vi "dotNETChart_DataChangeEvent.vi"(9 "Chart Settings clstr":T1={"Enable Mouse Zoom (only works in 2D mode)"=TRUE, "Chart Wall Transparency Level"=37, "Chart Wall Colour"=0, "x axis label"="X axis title", "y axis label"="Y axis title", "Enable3D"=TRUE, "3D Settings"={"Inclination"=20, "LightStyle"=2, "Perspective"=4, "WallWidth"=5, "Rotation"=25}, "BackGradientStyle"=2, "SkinStyle"=1, "Chart Background Gradient Colour"=0, "Chart Border Colour"=0, "Palette"=12, "LegendStyle"=0, "ChartType"=[10, 13], "SeriesDataColour"=[]} {"ChartType" items=["Point", "FastPoint", "Bubble", "Line", "Spline", "StepLine", "FastLine", "Bar", "StackedBar", "StackedBar100", "Column", "StackedColumn", "StackedColumn100", "Area", "SplineArea", "StackedArea", "StackedArea100", "Pie", "Doughnut", "Stock", "Candlestick", "Range", "SplineRange", "RangeBar", "RangeColumn", "Radar", "Polar", "ErrorBar", "BoxPlot", "Renko", "ThreeLineBreak", "Kagi", "PointAndFigure", "Funnel", "Pyramid"]; "LegendStyle" items=["Column", "Row", "Table"]; "Palette" items=["None", "Bright", "Grayscale", "Excel", "Light", "Pastel", "EarthTones", "SemiTransparent", "Berry", "Chocolate", "Fire", "SeaGreen", "BrightPastel"]; "SkinStyle" items=["None", "Emboss", "Raised", "Sunken", "FrameThin1", "FrameThin2", "FrameThin3", "FrameThin4", "FrameThin5", "FrameThin6", "FrameTitle1", "FrameTitle2", "FrameTitle3", "FrameTitle4", "FrameTitle5", "FrameTitle6", "FrameTitle7", "FrameTitle8"]; "BackGradientStyle" items=["None", "LeftRight", "TopBottom", "Center", "DiagonalLeft", "DiagonalRight", "HorizontalCenter", "VerticalCenter"]; "3D Settings"."LightStyle" items=["None", "Simplistic", "Realistic"]}, 10 "Microsoft Chart":refnum<k24>, 11 "chart data":dynamicdata(graph) caption="Chart Data") -> (0 "error out":errorcluster, 2 "reference out":refnum<k24>)   [LabVIEW 2013, in "dotNETChart XControl.xctl"]
uses:
  dotNETChart XControl.xctl
  System.Windows.Forms.DataVisualization
  typedefs/ChartSettings cluster.ctl
  typedefs/3DSettings.ctl
  typedefs/BackGradientStyle.ctl
  typedefs/SkinStyle.ctl
  typedefs/Palette.ctl
  typedefs/LegendStyle.ctl
  typedefs/ChartType.ctl
  System.Drawing
  <vilib>/express/express shared/transition.llb/Dynamic To Waveform Array.vi
  <vilib>/express/express signal manip/GetorSetDDTAttributes/Get DDT Attributes/Get DDT Properties.xnode
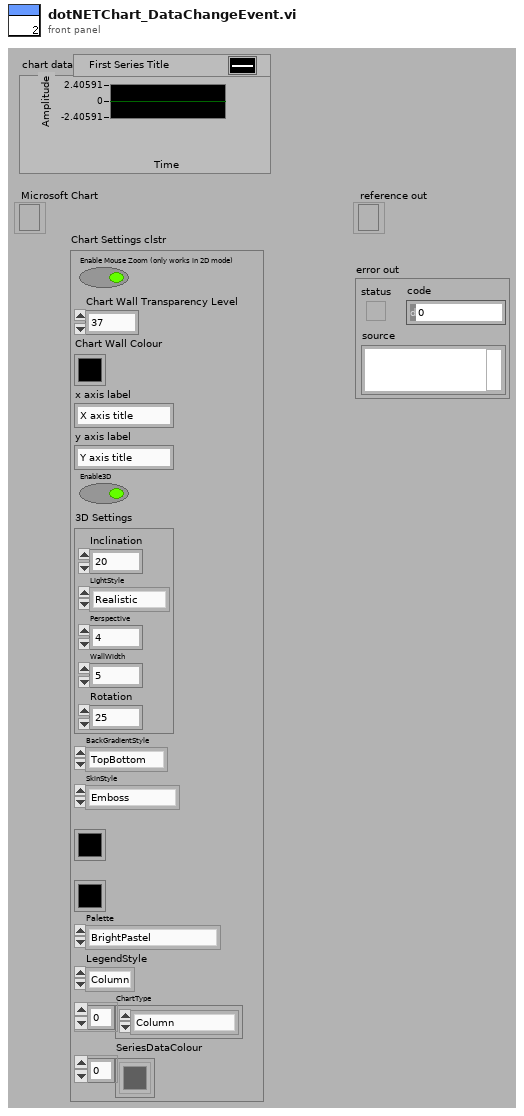
[diagram p1: front panel]
types:
  T1 = typedef "ChartSettings cluster.ctl" = cluster{"Enable Mouse Zoom (only works in 2D mode)":bool, "Chart Wall Transparency Level":i32, "Chart Wall Colour":u32, "x axis label":string, "y axis label":string, "Enable3D":bool, "3D Settings":T2, "BackGradientStyle":T3, "SkinStyle":T4, "Chart Background Gradient Colour":u32, "Chart Border Colour":u32, "Palette":T5, "LegendStyle":T6, "ChartType":T7[], "SeriesDataColour":u32[]}
  T2 = typedef "3DSettings.ctl" = cluster{"Inclination":i32, "LightStyle":i32, "Perspective":i32, "WallWidth":i32, "Rotation":i32}
  T3 = typedef "BackGradientStyle.ctl" = i32
  T4 = typedef "SkinStyle.ctl" = i32
  T5 = typedef "Palette.ctl" = i32
  T6 = typedef "LegendStyle.ctl" = i32
  T7 = typedef "ChartType.ctl" = i32
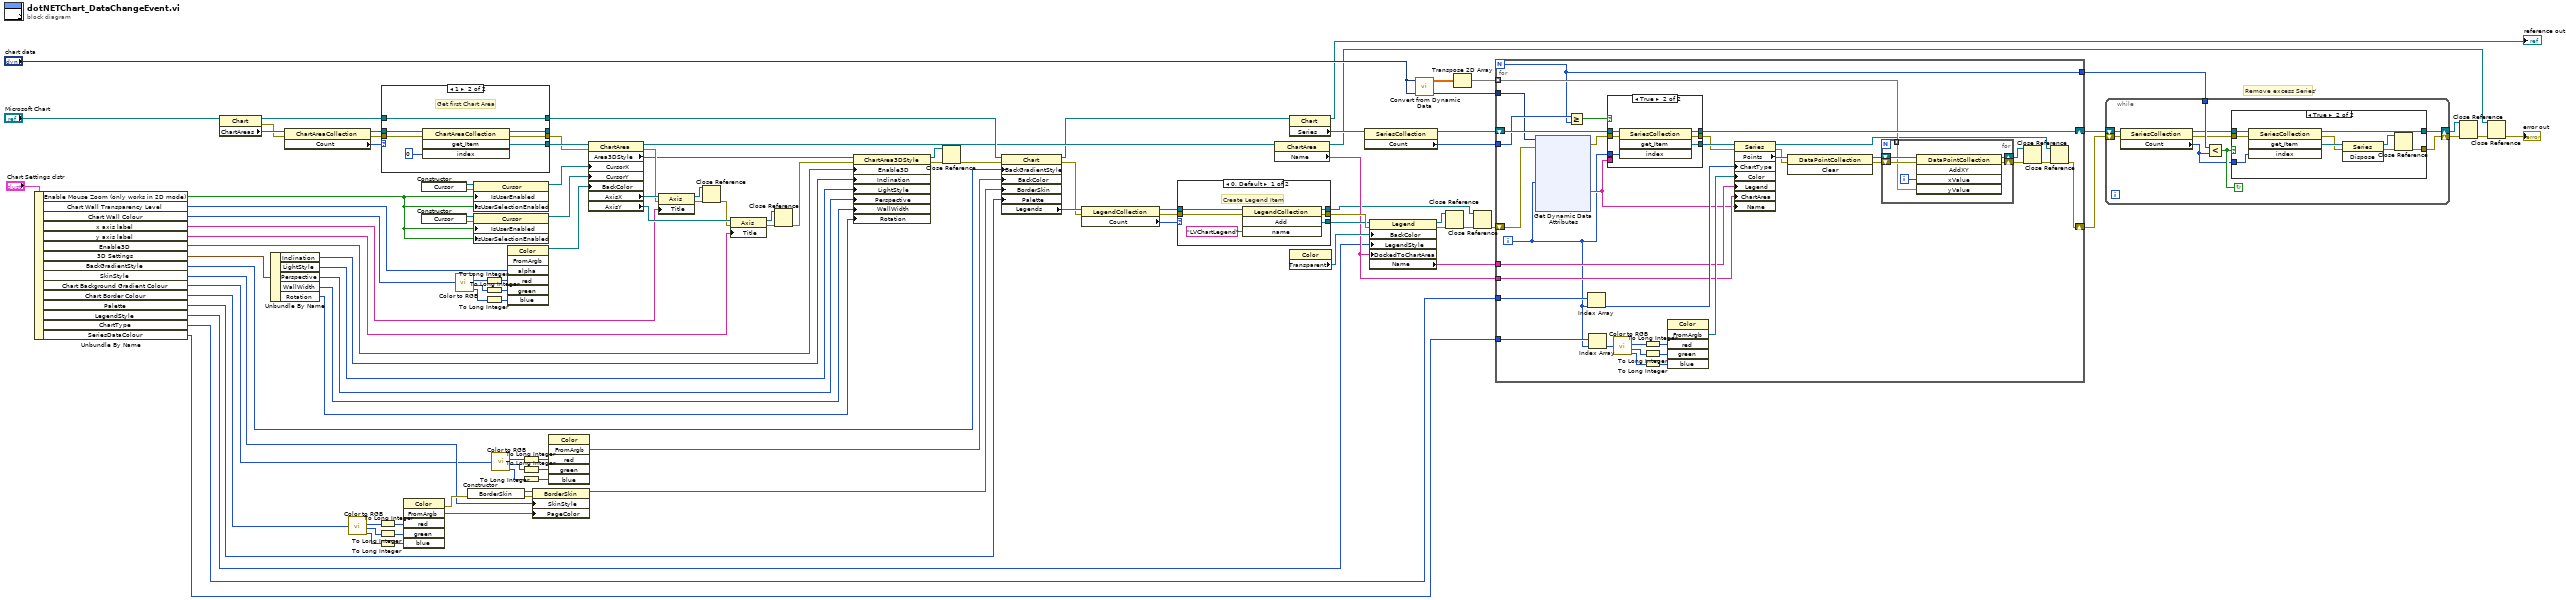
[diagram p0: block diagram]
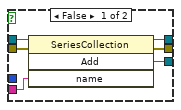
[diagram p3: hidden frame]
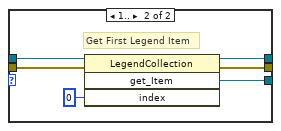
[diagram p4: hidden frame]
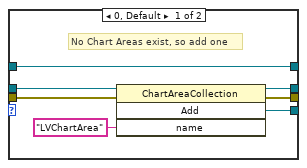
[diagram p5: hidden frame]
diagram:
  # "Remove excess Series'"
  n1 = Unbundle By Name("Chart Settings clstr") -> ("Enable Mouse Zoom (only works in 2D mode)"=w21:bool, "Chart Wall Transparency Level"=w20:i32, "Chart Wall Colour"=w19:u32, "x axis label"=w18:string, "y axis label"=w17:string, "Enable3D"=w16:bool, "3D Settings"=w10:T2, "BackGradientStyle"=w9:T3, "SkinStyle"=w8:T4, "Chart Background Gradient Colour"=w7:u32, "Chart Border Colour"=w6:u32, "Palette"=w5:T5, "LegendStyle"=w4:T6, "ChartType"=w3:T7[], "SeriesDataColour"=w2:u32[])
  n2 = property class="Chart"(reference="Microsoft Chart") -> (reference out=w101:refnum<k24>, error out=w105:errorcluster, "ChartAreas"=w106:refnum<k24>)  [unwired: 1 in]
  n3 = Unbundle By Name(w10) -> ("Inclination"=w15:i32, "LightStyle"=w14:i32, "Perspective"=w13:i32, "WallWidth"=w12:i32, "Rotation"=w11:i32)
  n4 = property class="ChartAreaCollection"(reference=w106, error in=w105) -> (reference out=w103:refnum<k24>, error out=w102:errorcluster, "Count"=w104:i32)
  n5 = call <vilib>:"Color to RGB.vi"("Color"=w6) -> ("R"=w32:u8, "G"=w33:u8, "B"=w34:u8)  [unwired: 1 out]
  n6 = To Long Integer(number=w32) -> (32bit integer=w31:i32)
  n7 = To Long Integer(number=w33) -> (32bit integer=w30:i32)
  n8 = To Long Integer(number=w34) -> (32bit integer=w29:i32)
  n9 = case shown="1" w104 {
    tunnel: w103 -> [w114 w121]
    tunnel: w102 -> [w113 w120]
    tunnel: [w111 w118] -> _
    tunnel: [w110 w117] -> w91
    tunnel: [w109 w116] -> w100
    tunnel: w101 -> [w108 w115]
    tunnel: [w108 w115] -> w73
    frame 0, Default {
      # "No Chart Areas exist, so add one"
      n10 = invoke class="ChartAreaCollection" method="Add"(reference=w114, error in=w113, "name"="LVChartArea") -> (reference out=w111:refnum<k24>, error out=w110:errorcluster, "Add"=w109:refnum<k24>)  [unwired: 1 in, 1 out]
    }
    frame 1 {
      # "Get first Chart Area"
      n11 = invoke class="ChartAreaCollection" method="get_Item"(reference=w121, error in=w120, "index"=0) -> (reference out=w118:refnum<k24>, error out=w117:errorcluster, "get_Item"=w116:refnum<k24>)  [unwired: 1 in, 1 out]
    }
  }
  n12 = invoke class="Color" method="FromArgb"("red"=w31, "green"=w30, "blue"=w29) -> (error out=w86:errorcluster, "FromArgb"=w85:refnum<k24>)  [unwired: 3 in, 4 out]
  n13 = constructor class="Cursor"() -> (reference out=w94:refnum<k24>, error out=w97:errorcluster)  [unwired: 3 in, 1 out]
  n14 = constructor class="Cursor"() -> (reference out=w98:refnum<k24>, error out=w99:errorcluster)  [unwired: 3 in, 1 out]
  n15 = call <vilib>:"Color to RGB.vi"("Color"=w19) -> ("R"=w40:u8, "G"=w39:u8, "B"=w38:u8)  [unwired: 1 out]
  n16 = constructor class="BorderSkin"(error in=w86) -> (reference out=w83:refnum<k24>, error out=w84:errorcluster)  [unwired: 2 in, 1 out]
  n17 = property class="Cursor"(reference=w94, error in=w97, "IsUserEnabled"=w21, "IsUserSelectionEnabled"=w21) -> (reference out=w96:refnum<k24>)  [unwired: 1 out]
  n18 = property class="Cursor"(reference=w98, error in=w99, "IsUserEnabled"=w21, "IsUserSelectionEnabled"=w21) -> (reference out=w95:refnum<k24>)  [unwired: 1 out]
  n19 = To Long Integer(number=w40) -> (32bit integer=w37:i32)
  n20 = To Long Integer(number=w39) -> (32bit integer=w36:i32)
  n21 = To Long Integer(number=w38) -> (32bit integer=w35:i32)
  n22 = call <vilib>:"Color to RGB.vi"("Color"=w7) -> ("R"=w28:u8, "G"=w27:u8, "B"=w26:u8)  [unwired: 1 out]
  n23 = invoke class="Color" method="FromArgb"("alpha"=w20, "red"=w37, "green"=w36, "blue"=w35) -> (reference out=w93:refnum<k24>)  [unwired: 3 in, 6 out]
  n24 = To Long Integer(number=w28) -> (32bit integer=w25:i32)
  n25 = To Long Integer(number=w27) -> (32bit integer=w24:i32)
  n26 = To Long Integer(number=w26) -> (32bit integer=w23:i32)
  n27 = property class="BorderSkin"(reference=w83, error in=w84, "SkinStyle"=w8, "PageColor"=w85) -> (reference out=w82:refnum<k24>)  [unwired: 1 out]
  n28 = invoke class="Color" method="FromArgb"("red"=w25, "green"=w24, "blue"=w23) -> ("FromArgb"=w87:refnum<k24>)  [unwired: 3 in, 5 out]
  n29 = property class="ChartArea"(reference=w100, error in=w91, "CursorX"=w96, "CursorY"=w95, "BackColor"=w93) -> (reference out=w72:refnum<k24>, error out=w90:errorcluster, "Area3DStyle"=w88:refnum<k24>, "AxisX"=w92:refnum<k24>, "AxisY"=w89:refnum<k24>)
  n30 = property class="Axis"(reference=w92, error in=w90, "Title"=w18) -> (reference out=w57:refnum<k24>, error out=w56:errorcluster)
  n31 = Close Reference(reference=w57, error in (no error)=w56) -> (error out=w55:errorcluster)
  n32 = property class="Axis"(reference=w89, error in=w55, "Title"=w17) -> (reference out=w53:refnum<k24>, error out=w54:errorcluster)
  n33 = Close Reference(reference=w53, error in (no error)=w54) -> (error out=w52:errorcluster)
  n34 = property class="ChartArea3DStyle"(reference=w88, error in=w52, "Enable3D"=w16, "Inclination"=w15, "LightStyle"=w14, "Perspective"=w13, "WallWidth"=w12, "Rotation"=w11) -> (reference out=w58:refnum<k24>, error out=w60:errorcluster)
  n35 = Close Reference(reference=w58, error in (no error)=w60) -> (error out=w59:errorcluster)
  n36 = property class="Chart"(reference=w73, error in=w59, "BackGradientStyle"=w9, "BackColor"=w87, "BorderSkin"=w82, "Palette"=w5) -> (reference out=w70:refnum<k24>, error out=w80:errorcluster, "Legends"=w81:refnum<k24>)
  n37 = property class="LegendCollection"(reference=w81, error in=w80) -> (reference out=w78:refnum<k24>, error out=w77:errorcluster, "Count"=w79:i32)
  n38 = case shown="0, Default" w79 {
    tunnel: w78 -> [w127 w131]
    tunnel: w77 -> [w126 w132]
    tunnel: [w124 w129] -> w75
    tunnel: [w123 w133] -> w76
    tunnel: [w122 w130] -> w47
    frame 0, Default {
      # "Create Legend Item"
      n39 = invoke class="LegendCollection" method="Add"(reference=w127, error in=w126, "name"="LVChartLegend") -> (reference out=w122:refnum<k24>, error out=w123:errorcluster, "Add"=w124:refnum<k24>)  [unwired: 1 in, 1 out]
    }
    frame 1.. {
      # "Get First Legend Item"
      n40 = invoke class="LegendCollection" method="get_Item"(reference=w131, error in=w132, "index"=0) -> (reference out=w130:refnum<k24>, error out=w133:errorcluster, "get_Item"=w129:refnum<k24>)  [unwired: 1 in, 1 out]
    }
  }
  n41 = property class="ChartArea"(reference=w72) -> (reference out=w43:refnum<k24>, "Name"=w66:string)  [unwired: 1 in, 1 out]
  n42 = property class="Chart"(reference=w70) -> (reference out=→"reference out":refnum<k24>, "Series"=w69:refnum<k24>)  [unwired: 1 in, 1 out]
  n43 = property class="Color"() -> ("Transparent"=w74:refnum<k24>)  [unwired: 2 in, 2 out]
  n44 = property class="SeriesCollection"(reference=w69) -> (reference out=w68:refnum<k24>, "Count"=w67:i32)  [unwired: 1 in, 1 out]
  n45 = property class="Legend"(reference=w75, error in=w76, "BackColor"=w74, "LegendStyle"=w4, "DockedToChartArea"=w66) -> (reference out=w50:refnum<k24>, error out=w51:errorcluster, "Name"=w65:string)
  n46 = call "Convert from Dynamic Data"("Dynamic Data Type"="chart data") -> ("Array"=w64:dbl[][])  [unwired: 3 in]
  n47 = Close Reference(reference=w50, error in (no error)=w51) -> (error out=w49:errorcluster)
  n48 = Transpose 2D Array(2D array=w64) -> (transposed array=w1:dbl[][])
  n49 = Close Reference(reference=w47, error in (no error)=w49) -> (error out=w48:errorcluster)
  n50 = for {
    N -> [w139]
    tunnel: "chart data" -> [w137]
    shift-right: [w140] -> w61
    shift-left: w48 -> [w136]
    shift-right: [w150] -> w63
    shift-left: w68 -> [w168]
    tunnel: w67 -> [w166]
    tunnel: w3 -> [w163]
    tunnel: w2 -> [w154]
    tunnel: w66 -> [w151]
    tunnel: w65 -> [w152]
    tunnel: w1 -> [w145] mode=indexing
    tunnel: [w139] -> w62
    i -> [w134]
    n51 = xnode "Get Dynamic Data Attributes"("Signal Index"=w134, "Signals In"=w137, "error in"=w136) -> ("Signal Name"=w138:string, "error out"=w135:errorcluster)  [unwired: 2 out]
    n52 = Greater Or Equal?(x=w166, y=w139) -> (x >= y?=w167:bool)
    n53 = Index Array(array=w163, index=w134) -> (element=w162:T7)
    n54 = Index Array(array=w154, index=w134) -> (element=w153:u32)
    n55 = case shown="True" w167 {
      tunnel: w168 -> [w179 w186]
      tunnel: w134 -> [_ w185]
      tunnel: [w177 w184] -> w165
      tunnel: [w180 w183] -> w164
      tunnel: [w178 w182] -> w150
      tunnel: w138 -> [w176 _]
      tunnel: w135 -> [w175 w181]
      frame False {
        n56 = invoke class="SeriesCollection" method="Add"(reference=w179, error in=w175, "name"=w176) -> (reference out=w178:refnum<k24>, error out=w180:errorcluster, "Add"=w177:refnum<k24>)  [unwired: 1 in, 1 out]
      }
      frame True {
        n57 = invoke class="SeriesCollection" method="get_Item"(reference=w186, error in=w181, "index"=w185) -> (reference out=w182:refnum<k24>, error out=w183:errorcluster, "get_Item"=w184:refnum<k24>)  [unwired: 1 in, 1 out]
      }
    }
    n58 = call <vilib>:"Color to RGB.vi"("Color"=w153) -> ("R"=w160:u8, "G"=w159:u8, "B"=w158:u8)  [unwired: 1 out]
    n59 = To Long Integer(number=w160) -> (32bit integer=w157:i32)
    n60 = To Long Integer(number=w159) -> (32bit integer=w156:i32)
    n61 = To Long Integer(number=w158) -> (32bit integer=w155:i32)
    n62 = invoke class="Color" method="FromArgb"("red"=w157, "green"=w156, "blue"=w155) -> ("FromArgb"=w161:refnum<k24>)  [unwired: 3 in, 5 out]
    n63 = property class="Series"(reference=w165, error in=w164, "ChartType"=w162, "Color"=w161, "Legend"=w152, "ChartArea"=w151, "Name"=w138) -> (reference out=w141:refnum<k24>, error out=w147:errorcluster, "Points"=w149:refnum<k24>)
    n64 = invoke class="DataPointCollection" method="Clear"(reference=w149, error in=w147) -> (reference out=w148:refnum<k24>, error out=w146:errorcluster)  [unwired: 1 in, 1 out]
    n65 = for {
      tunnel: w145 -> [w172] mode=indexing
      shift-right: [w170] -> w143
      shift-left: w148 -> [w174]
      shift-right: [w169] -> w144
      shift-left: w146 -> [w173]
      i -> [w171]
      n66 = invoke class="DataPointCollection" method="AddXY"(reference=w174, error in=w173, "xValue"=w171, "yValue"=w172) -> (reference out=w170:refnum<k24>, error out=w169:errorcluster)  [unwired: 1 in, 3 out]
    }
    n67 = Close Reference(reference=w143, error in (no error)=w144) -> (error out=w142:errorcluster)
    n68 = Close Reference(reference=w141, error in (no error)=w142) -> (error out=w140:errorcluster)
  }
  n69 = while {
    tunnel: w62 -> [w208]
    shift-right: [w201] -> w46
    shift-left: w61 -> [w205]
    shift-right: [w202] -> w45
    shift-left: w63 -> [w209]
    stop <- w204 continue-if-true
    n70 = property class="SeriesCollection"(reference=w209, error in=w205) -> (reference out=w207:refnum<k24>, error out=w206:errorcluster, "Count"=w203:i32)
    n71 = Less?(x=w208, y=w203) -> (x < y?=w204:bool)
    n72 = case shown="True" w204 {
      tunnel: w207 -> [w210 w220]
      tunnel: w206 -> [w211 w219]
      tunnel: w203 -> [_ w218]
      tunnel: [w210 w213] -> w202
      tunnel: [w211 w212] -> w201
      frame False {
      }
      frame True {
        n73 = invoke class="SeriesCollection" method="get_Item"(reference=w220, error in=w219, "index"=w218) -> (reference out=w213:refnum<k24>, error out=w216:errorcluster, "get_Item"=w217:refnum<k24>)  [unwired: 1 in, 1 out]
        n74 = invoke class="Series" method="Dispose"(reference=w217, error in=w216) -> (reference out=w214:refnum<k24>, error out=w215:errorcluster)  [unwired: 1 in, 1 out]
        n75 = Close Reference(reference=w214, error in (no error)=w215) -> (error out=w212:errorcluster)
      }
    }
  }
  n76 = Close Reference(reference=w45, error in (no error)=w46) -> (error out=w44:errorcluster)
  n77 = Close Reference(reference=w43, error in (no error)=w44) -> (error out=→"error out":errorcluster)
